vi "Update Account file.vi"(8 "error in (no error)":errorcluster, 9 "Account":string, 10 "Balance":dbl, 11 "name or relative path":path=path "ATM accounts.txt") -> (0 "error out":errorcluster)   [LabVIEW 2020]
uses:
  <vilib>/Utility/file.llb/Read Delimited Spreadsheet (string).vi
  <vilib>/Utility/file.llb/Write Delimited Spreadsheet (string).vi
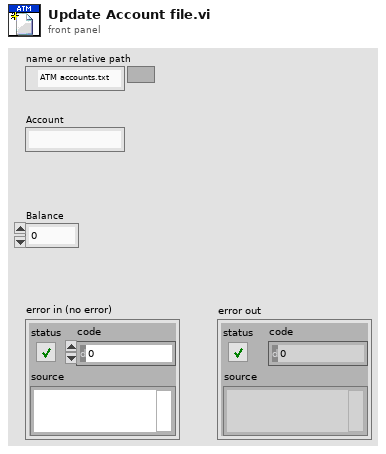
[diagram p1: front panel]
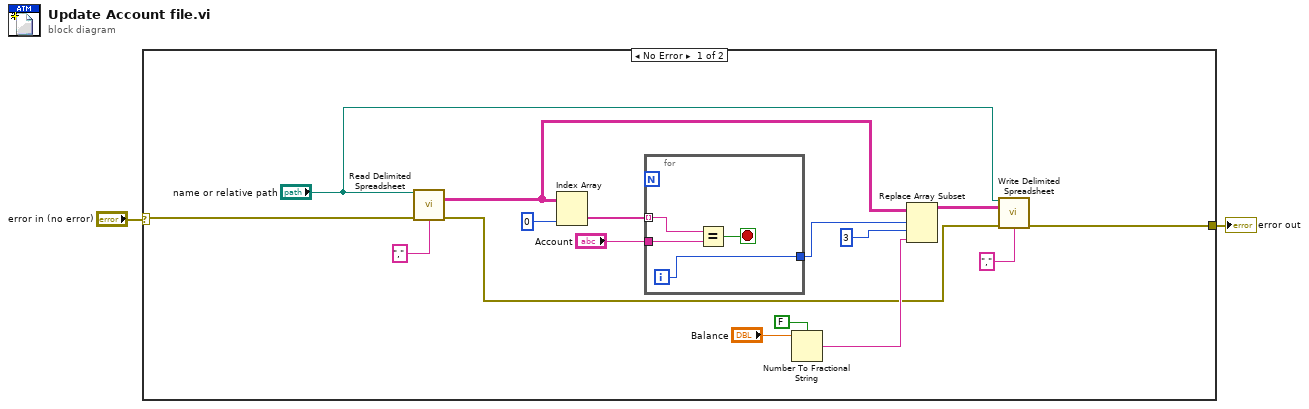
[diagram p0: block diagram]
diagram:
  n1 = case shown="No Error" "error in (no error)" {
    selector: "error in (no error)" -> [w4 w23]
    tunnel: [w5 w23] -> w1
    frame No Error {
      n2 = call-poly <vilib>:"Read Delimited Spreadsheet.vi"("file path (dialog if empty)"="name or relative path", "error in (no error)"=w4, "delimiter (\\t)"="," ("delimiter (\\t)")) -> ("all rows"=w15:string[][], "error out"=w6:errorcluster)  [unwired: 7 in, 4 out]
      n3 = Index Array(array=w15, index (col)=0 ("disabled index (col)")) -> (element=w16:string[])  [unwired: 1 in]
      n4 = for {
        tunnel: "Account" -> [w22]
        tunnel: w16 -> [w20] mode=indexing
        tunnel: [w19] -> w14
        i -> [w19]
        stop <- w21 stop-if-true
        n5 = Equal?(x=w20, y=w22) -> (x = y?=w21:bool)
      }
      n6 = Number To Fractional String(use system decimal point (T)=FALSE, number="Balance") -> (F-format string=w10:string)  [unwired: 2 in]
      n7 = Replace Array Subset(array=w15, new element=w10, index (row)=w14, index (col)=3 ("disabled index (col)")) -> (w8:string[][])
      n8 = call-poly <vilib>:"Write Delimited Spreadsheet.vi"("file path (dialog if empty)"="name or relative path", "2D data"=w8, "error in (no error)"=w6, "delimiter (\\t)"="," ("delimiter (\\t)")) -> ("error out"=w5:errorcluster)  [unwired: 10 in, 1 out]
    }
    frame Error {
    }
  }
  "error out" <- w1
